vi "pumping station.vi"() -> ()   [LabVIEW 2023]
panel:
  out "Level":dbl
  in  "Set Point":dbl
  out "Low":bool
  out "Adequate":bool
  out "High":bool
  out "Tank-4":dbl(slide) scale=0.0..1000.0
  out "Low":bool
  out "Adequate 2":bool
  out "High":bool
  out "Tank-3":dbl(slide) scale=0.0..1000.0
  out "Low":bool
  out "Adequate":bool
  out "High":bool
  out "Tank-2":dbl(slide) scale=0.0..1000.0
  out "Low":bool
  out "Adequate":bool
  out "High":bool
  out "Tank-1":dbl(slide) scale=0.0..1000.0
  out "Adequate":bool
  out "Waveform Chart":u32(graph) caption="Water Filling Status"
  out "Low":bool
  out "High":bool
  out "Reservoir":dbl(slide) scale=0.0..10000.0
  in  "Delay":dbl(knob) scale=0.0..10.0
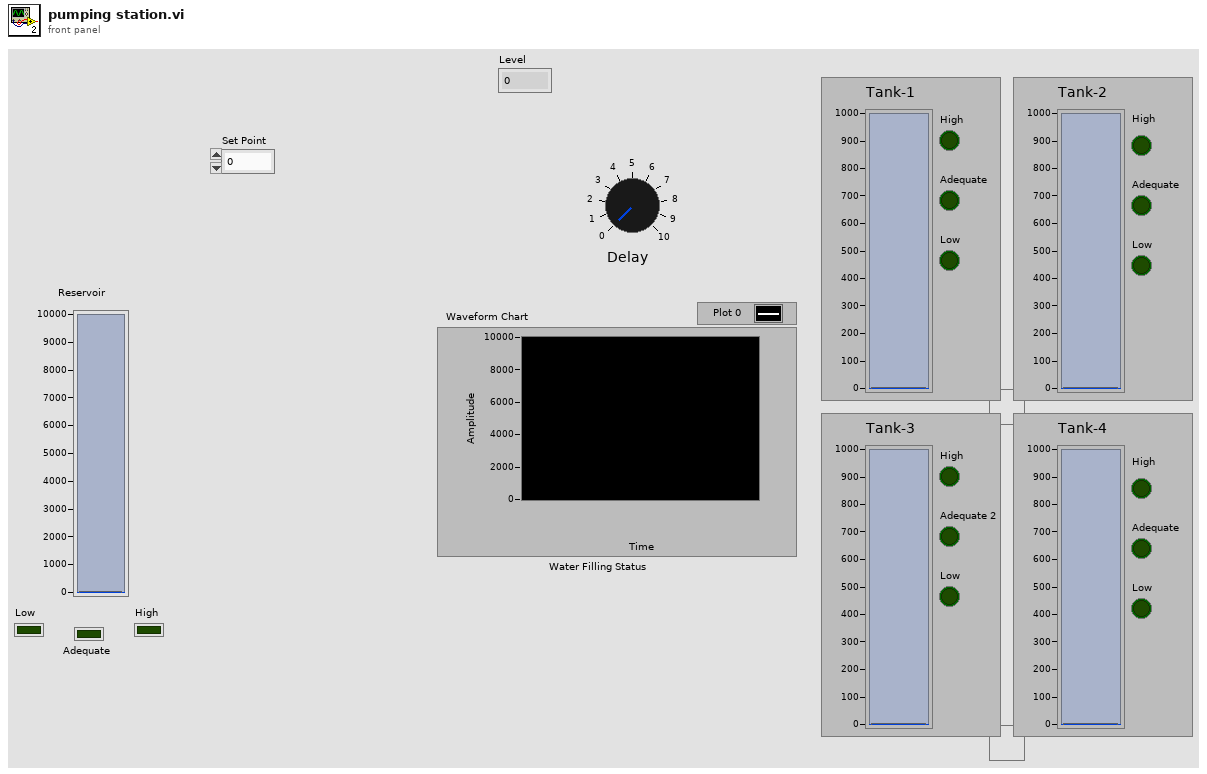
[diagram p1: front panel]
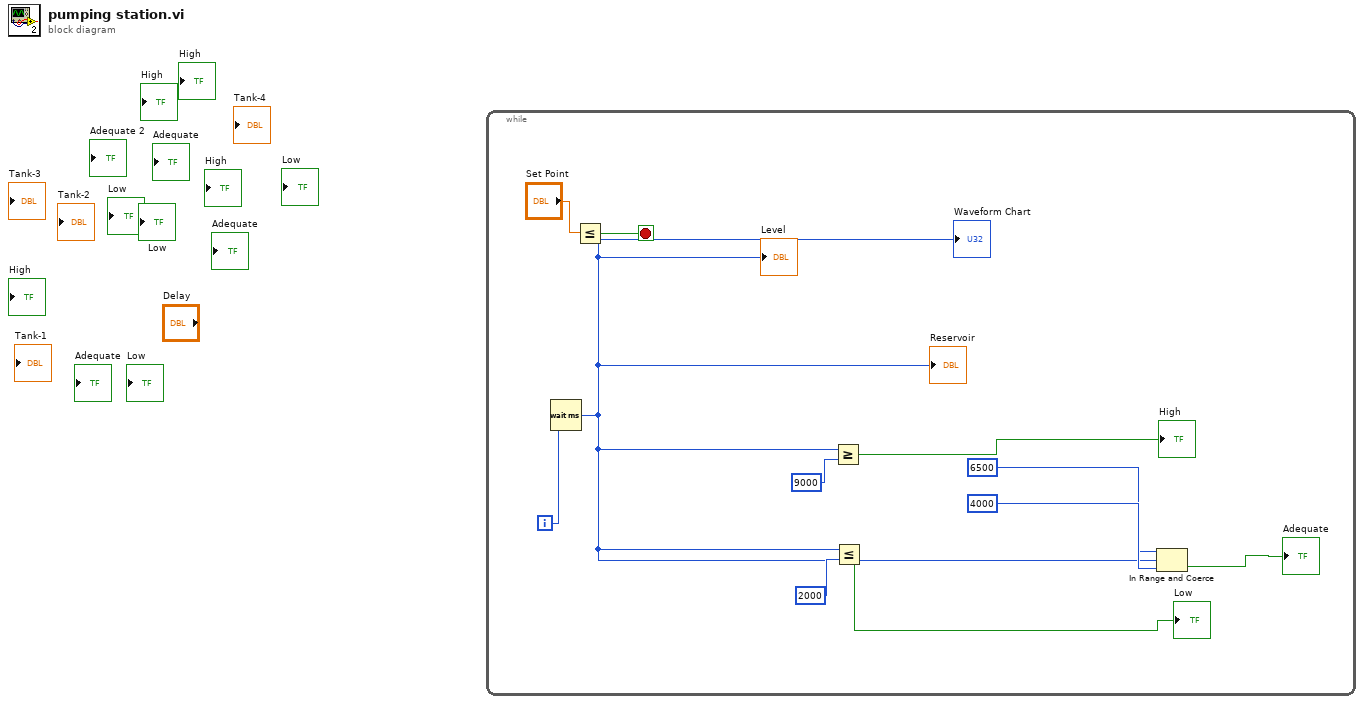
[diagram p0: block diagram]
diagram:
  n1 = while {
    i -> [w2]
    stop <- w4 stop-if-true
    n2 = Wait (ms)(milliseconds to wait=w2) -> (millisecond timer value=w1:u32)
    "Reservoir" <- w1
    "Waveform Chart" <- w1
    "Level" <- w1
    n3 = Less Or Equal?(x="Set Point", y=w1) -> (x <= y?=w4:bool)
    n4 = Greater Or Equal?(x=w1, y=9000) -> (x >= y?=→"High":bool)
    n5 = Less Or Equal?(x=w1, y=2000) -> (x <= y?=→"Low":bool)
    n6 = In Range and Coerce(upper limit=6500, x=w1, lower limit=4000) -> (In Range?=→"Adequate":bool)  [unwired: 1 out]
  }
